vi "Generate Simulated Data.vi"(6 "Acquisition":refnum<queue>, 8 "error in (no error)":errorcluster, 10 "Longueur d'onde":dbl) -> (0 "error out":errorcluster, 2 "Data Out":variant[](array[variant]), 3 "Disconnected":bool=TRUE)   [LabVIEW 2022 SP3, in "Acquisition.lvlib"]
doc: "Generates sample waveforms according to the signal type in the HW Config input."
uses:
  Acquisition.lvlib
  support/Message Queue/Message Cluster.ctl
  <vilib>/DAQmx/write.llb/DAQmx Write (Digital 1D Bool NChan 1Samp 1Line).vi
  <vilib>/numeric/Random Number (Range) U64.vi
  <vilib>/DAQmx/read.llb/DAQmx Read (Analog 1D Wfm NChan NSamp).vi
  <vilib>/Analysis/baseanly.llb/Mean (DBL).vi
  <vilib>/numeric/sub_Random U32.vi
  <vilib>/DAQmx/create/channels.llb/DAQmx Create Channel (DO-Digital Output).vi
  <vilib>/DAQmx/miscellaneous.llb/DAQmx Fill In Error Info.vi
  <vilib>/DAQmx/create/channels.llb/DAQmx Create Channel (AI-Voltage-Basic).vi
  <vilib>/DAQmx/configure/timing.llb/DAQmx Timing (Sample Clock).vi
  support/Message Queue/Enqueue Message (Single).vi
  GlobalVariable/GlobalPowerByTime.vi
  GlobalVariable/GlobalSet0.vi
  GlobalVariable/GlobalPosYbyTime.vi
  GlobalVariable/GlobalPosXbyTime.vi
  GlobalVariable/GlobalProfileByTime.vi
  GlobalVariable/Globalt0.vi
  GlobalVariable/GlobalTimeStep.vi
  <vilib>/gmath/interp.llb/Create Mesh Grid (2D) (x,y arrays).vi
  <vilib>/Analysis/2dsp.llb/2D Convolution (DBL).vi
  <vilib>/Analysis/NI_AALBase.lvlib
  support/Message Queue/Message Queue.lvlib
  <vilib>/gmath/NI_Gmath.lvlib
  <vilib>/Analysis/NI_AALPro.lvlib
  <resource>/objmgr/daqmx.rc
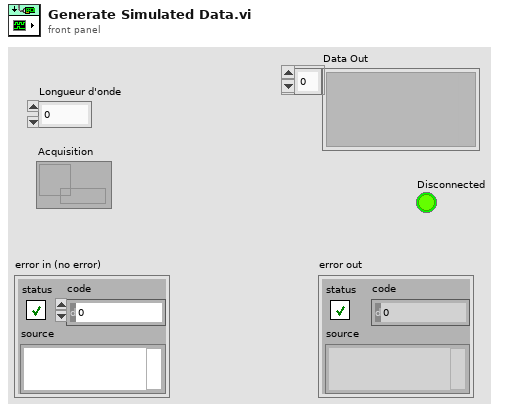
[diagram p1: front panel]
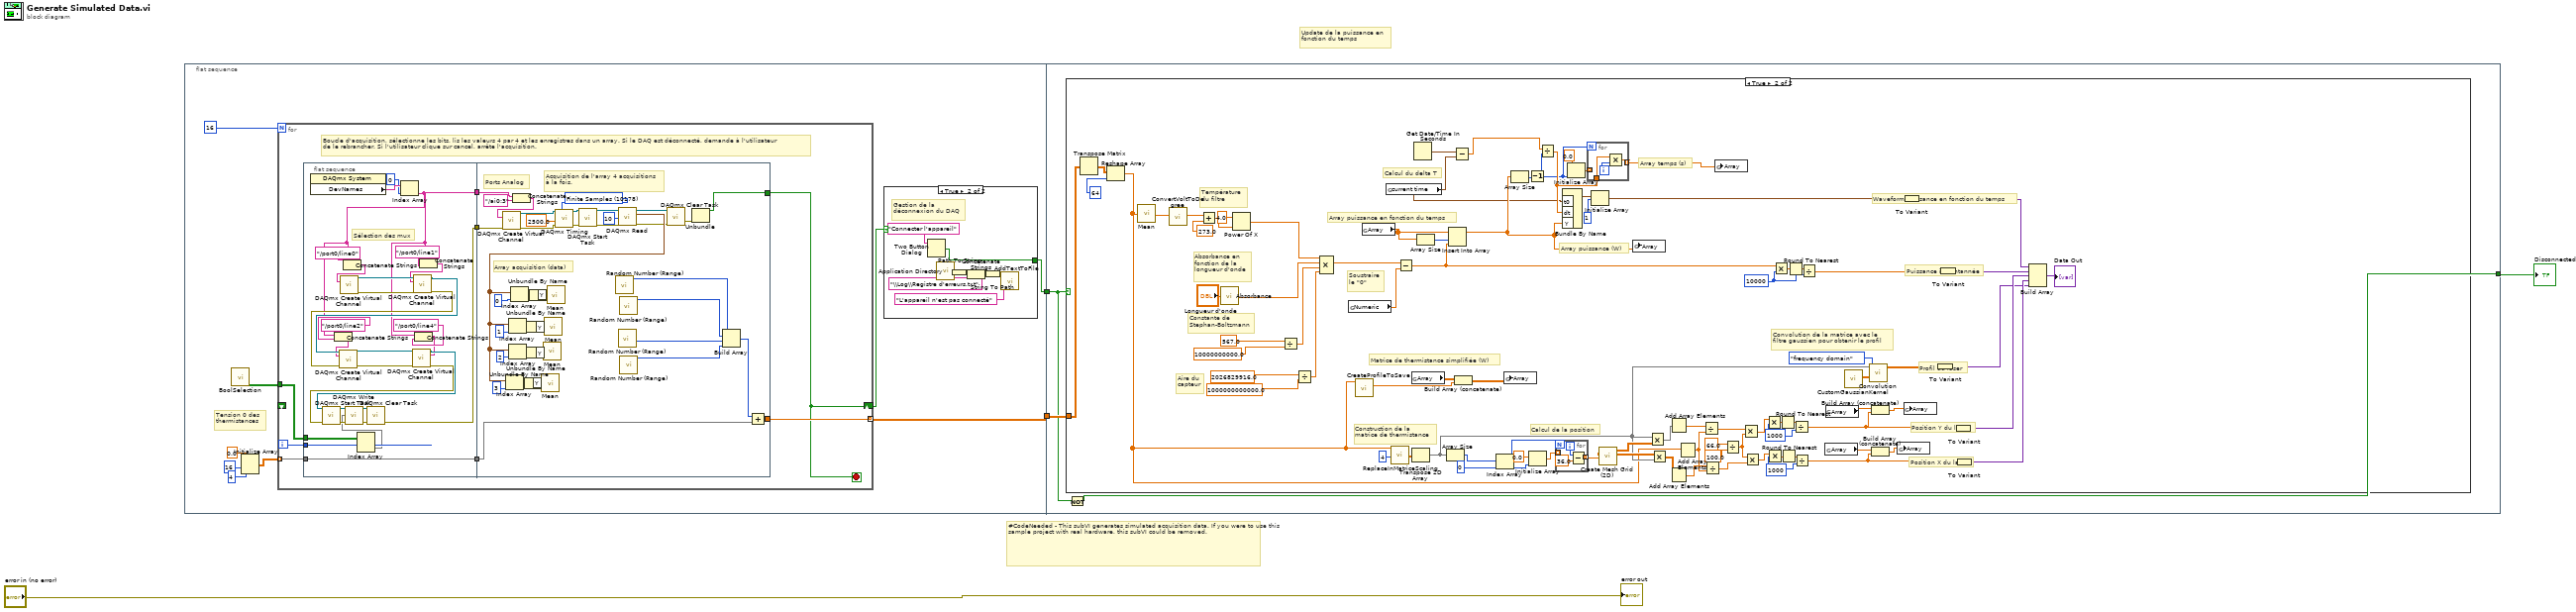
[diagram p0: block diagram]
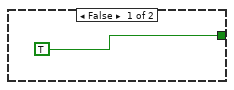
[diagram p2: hidden frame]
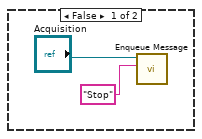
[diagram p3: hidden frame]
diagram:
  # "Update de la puissance en\nfonction du temps"
  # "#CodeNeeded - This subVI generates simulated acquisition data. If you were to use this sample project with real hardware, this subVI could be removed."
  n1 = flat-sequence {
    tunnel: [w11] -> w3
    tunnel: [w10] -> w2
    tunnel: w3 -> [w98]
    tunnel: w2 -> [w97]
    tunnel: [w96] -> w1
    frame #0 {
      # "Tension 0 des \nthermistances"
      n2 = call "BoolSelection.vi"() -> ("BoolSelection"=w12:bool[][])  [unwired: 11 in]
      n3 = Initialize Array(0.0 ("element"), 16 ("dimension size"), 4 ("dimension size")) -> (w6:dbl[][])
      n4 = for {
        N: 16 -> [_]
        tunnel: w12 -> [w28]
        tunnel: w6 -> [w26] mode=indexing
        tunnel: [w25] -> w11 mode=indexing
        shift-right: [w24] -> w5
        shift-left: _ -> [_]
        i -> [w29]
        stop <- w24 stop-if-true
        # "Boucle d'acquisition, sélectionne les bits, lis les valeurs 4 par 4 et les enregistres dans un array. Si le DAQ est déconnecté, demande à l'utilisateur \nde le rebrancher. Si l'utilisateur clique sur cancel, arrête l'acquisition."
        n5 = flat-sequence {
          tunnel: w29 -> [w44]
          tunnel: [w55] -> w30
          tunnel: w28 -> [w43]
          tunnel: [w42] -> w27
          tunnel: w26 -> [w42]
          tunnel: [w31] -> w23
          tunnel: w30 -> [w87]
          tunnel: w27 -> [w62]
          tunnel: [w64] -> w25
          tunnel: [w69] -> w24
          tunnel: w23 -> [w59]
          frame #0 {
            # "Sélection des mux"
            n6 = property class="DAQmx System"() -> ("DevNames"=w41:tag[])  [unwired: 2 in, 2 out]
            n7 = Index Array(array=w43, index (row)=w44) -> (element=w56:bool[])  [unwired: 1 in]
            n8 = Index Array(array=w41, index=0) -> (element=w31:tag)
            n9 = Concatenate Strings(w31, "/port0/line2" ("string")) -> (w34:string)
            n10 = Concatenate Strings(w31, "/port0/line0" ("string")) -> (w39:string)
            n11 = call-poly <vilib>:"DAQmx Create Virtual Channel.vi"("lines"=w39) -> ("task out"=w51:refnum<k21>, "error out"=w52:errorcluster)  [unwired: 13 in]
            n12 = Concatenate Strings(w31, "/port0/line4" ("string")) -> (w32:string)
            n13 = Concatenate Strings(w31, "/port0/line1" ("string")) -> (w36:string)
            n14 = call-poly <vilib>:"DAQmx Create Virtual Channel.vi"("task in"=w51, "lines"=w36, "error in"=w52) -> ("task out"=w50:refnum<k21>, "error out"=w49:errorcluster)  [unwired: 11 in]
            n15 = call-poly <vilib>:"DAQmx Create Virtual Channel.vi"("task in"=w50, "lines"=w34, "error in"=w49) -> ("task out"=w47:refnum<k21>, "error out"=w48:errorcluster)  [unwired: 11 in]
            n16 = call-poly <vilib>:"DAQmx Create Virtual Channel.vi"("task in"=w47, "lines"=w32, "error in"=w48) -> ("task out"=w46:refnum<k21>, "error out"=w45:errorcluster)  [unwired: 11 in]
            n17 = call <vilib>:"DAQmx Start Task.vi"("task/channels in"=w46, "error in"=w45) -> ("task out"=w57:refnum<k21>, "error out"=w58:errorcluster)  [unwired: 12 in]
            n18 = call-poly <vilib>:"DAQmx Write.vi"("task/channels in"=w57, "data"=w56, "error in"=w58) -> ("task out"=w54:refnum<k21>, "error out"=w53:errorcluster)  [unwired: 10 in, 1 out]
            n19 = call <vilib>:"DAQmx Clear Task.vi"("task in"=w54, "error in"=w53) -> ("error out"=w55:errorcluster)  [unwired: 13 in]
          }
          frame #1 {
            w89 = 10178 items=["Finite Samples"=10178, "Continuous Samples"=10123, "Hardware Timed Single Point"=12522] ("sample mode")
            # "Ports Analog"
            # "Array acquisition (data)"
            # "Acquisition de l'array 4 acquisitions\nà la fois."
            n20 = Concatenate Strings(w59, "/ai0:3" ("string")) -> (w60:string)
            n21 = call-poly <vilib>:"DAQmx Create Virtual Channel.vi"("physical channels"=w60, "error in"=w87) -> ("task out"=w94:refnum<k21>, "error out"=w93:errorcluster)  [unwired: 12 in]
            n22 = call-poly <vilib>:"DAQmx Timing.vi"("task/channels in"=w94, "sample mode"=w89, "rate"=2500.0, "error in"=w93) -> ("task out"=w90:refnum<k21>, "error out"=w91:errorcluster)  [unwired: 10 in]
            n23 = call <vilib>:"DAQmx Start Task.vi"("task/channels in"=w90, "error in"=w91) -> ("task out"=w92:refnum<k21>, "error out"=w95:errorcluster)  [unwired: 12 in]
            n24 = call-poly <vilib>:"Random Number (Range).vi"() -> ("number"=w67:u64)  [unwired: 11 in]
            n25 = call-poly <vilib>:"Random Number (Range).vi"() -> ("number"=w65:u64)  [unwired: 11 in]
            n26 = call-poly <vilib>:"DAQmx Read.vi"("task/channels in"=w92, "number of samples per channel"=10, "error in"=w95) -> ("task out"=w71:refnum<k21>, "data"=w80:waveform(dbl)[], "error out"=w70:errorcluster)  [unwired: 10 in]
            n27 = Index Array(array=w80, index=3) -> (element=w76:waveform(dbl))
            n28 = Index Array(array=w80, index=1) -> (element=w78:waveform(dbl))
            n29 = Index Array(array=w80, index=2) -> (element=w77:waveform(dbl))
            n30 = Index Array(array=w80, index=0) -> (element=w79:waveform(dbl))
            n31 = Unbundle By Name(w76) -> ("Y"=w72:dbl[])
            n32 = Unbundle By Name(w78) -> ("Y"=w74:dbl[])
            n33 = Unbundle By Name(w77) -> ("Y"=w73:dbl[])
            n34 = Unbundle By Name(w79) -> ("Y"=w75:dbl[])
            n35 = call-poly <vilib>:"Mean.vi"("X"=w72) -> ()  [unwired: 2 out]
            n36 = call-poly <vilib>:"Mean.vi"("X"=w73) -> ()  [unwired: 2 out]
            n37 = call-poly <vilib>:"Mean.vi"("X"=w74) -> ()  [unwired: 2 out]
            n38 = call-poly <vilib>:"Mean.vi"("X"=w75) -> ()  [unwired: 2 out]
            n39 = call-poly <vilib>:"Random Number (Range).vi"() -> ("number"=w68:u64)  [unwired: 11 in]
            n40 = call-poly <vilib>:"Random Number (Range).vi"() -> ("number"=w66:u64)  [unwired: 11 in]
            n41 = call <vilib>:"DAQmx Clear Task.vi"("task in"=w71, "error in"=w70) -> ("error out"=w85:errorcluster)  [unwired: 13 in]
            n42 = Unbundle(w85) -> ("status"=w69:bool)  [unwired: 2 out]
            n43 = Build Array(w67, w68, w65, w66) -> (w63:u64[])
            n44 = Add(x=w63, y=w62) -> (x+y=w64:dbl[])
          }
        }
      }
      n45 = case shown="True" w5 {
        tunnel: [TRUE w22] -> w10
        frame False {
        }
        frame True {
          # "Gestion de la \ndéconnexion du DAQ"
          n46 = Two Button Dialog(message="Connecter l'appareil") -> (T button?=w22:bool)  [unwired: 2 in]
          n47 = call <vilib>:"Application Directory.vi"() -> ("Application Directory"=w19:path)
          n48 = Path To String(path=w19) -> (string=w20:string)
          n49 = Concatenate Strings(w20, "\\Log\\Registre d'erreurs.txt") -> (w21:string)
          n50 = String To Path(string=w21) -> (path=w17:path)
          n51 = call "AddTextToFile.vi"("Ajouter du texte"="L'appareil n'est pas connecté", "Fichier"=w17) -> ()  [unwired: 10 in]
        }
      }
    }
    frame #1 {
      n52 = case shown="True" w97 {
        tunnel: w98 -> [_ w122]
        frame False {
          n53 = call-poly "Enqueue Message.vi"("Message"="Stop", "Message Queue"="Acquisition") -> ()  [unwired: 8 in, 2 out]
        }
        frame True {
          w136 = 1000
          w140 = 1000
          w146 = 10000
          # "Calcul du delta T"
          # "Matrice de thermistance simplifiée (W)"
          # "Soustraire\nle \"0\""
          # "Constante de \nStephan-Boltzmann"
          # "Absorbance en\nfonction de la \nlongueur d'onde"
          # "Température \ndu filtre"
          # "Aire du\ncapteur"
          # "Calcul de la position"
          # "Construction de la \nmatrice de thermistance"
          # "Position X du laser"
          # "Position Y du laser"
          # "Profil du laser"
          # "Puissance instantannée"
          # "Waveform puissance en fonction du temps"
          # "Array puissance (W)"
          # "Array temps (s)"
          # "Convolution de la matrice avec le \nfiltre gaussien pour obtenir le profil"
          # "Array puissance en fonction du temps"
          n54 = Transpose Matrix(1:w122) -> (0:w123:dbl[][])
          n55 = Reshape Array(w123, 64 ("dimension size")) -> (w117:dbl[])
          n56 = call-poly <vilib>:"Mean.vi"("X"=w117) -> ("mean"=w130:dbl)  [unwired: 1 out]
          n57 = call "ConvertVoltToDegree.vi"("Tension"=w130) -> ("Température"=w129:dbl)  [unwired: 10 in]
          n58 = Add(x=w129, y=273.0) -> (x+y=w175:dbl)
          n59 = call "Absorbance.vi"("Longueur d'onde"="Longueur d'onde") -> ("absorbance"=w126:dbl)  [unwired: 10 in]
          n60 = Power Of X(1:w175, 2:4.0 ("y")) -> (0:w125:dbl)
          n61 = Divide(x=567.0, y=10000000000.0) -> (x/y=w127:dbl)
          n62 = Divide(x=2026829916.0, y=1000000000000.0) -> (x/y=w128:dbl)
          n63 = Compound Arithmetic op=MULTIPLY(w125, w126, w127, w128) -> (w121:dbl)
          n64 = global read "GlobalSet0.vi" "Numeric"() -> (w120:dbl)
          n65 = call "CreateProfileToSave.vi"("Input Array"=w117) -> ("Ouput array"=w107:dbl[])  [unwired: 10 in]
          n66 = global read "GlobalPowerByTime.vi" "Array"() -> (w187:dbl[])
          n67 = global read "Globalt0.vi" "current time"() -> (w102:timestamp)
          n68 = call "ReplaceInMatriceScaling.vi"("Input Scaling"=4, "Input Array"=w117) -> ("Output Array"=w182:dbl[][])  [unwired: 9 in]
          n69 = Subtract(x=w121, y=w120) -> (x-y=w119:dbl)
          n70 = global read "GlobalProfileByTime.vi" "Array"() -> (w106:dbl[][])
          n71 = Transpose 2D Array(2D array=w182) -> (transposed array=w118:dbl[][])
          n72 = Get Date/Time In Seconds() -> (seconds since 1Jan1904=w103:timestamp)
          n73 = Array Size(array=w187) -> (size(s)=w186:i32)
          n74 = Array Size(array=w118) -> (size(s)=w169:i32[])
          n75 = Insert Into Array(array=w187, index=w186, new element=w119) -> (w116:dbl[])
          n76 = Subtract(x=w103, y=w102) -> (x-y=w101:dbl)
          n77 = Build Array (concatenate)(w106, w107) -> (w108:dbl[][])
          n78 = Index Array(array=w169, index=0) -> (element=w164:i32)
          n79 = global write "GlobalProfileByTime.vi" "Array"(w108) -> ()
          n80 = Array Size(array=w116) -> (size(s)=w105:i32)
          n81 = Decrement(x=w105) -> (x-1=w104:i32)
          n82 = Initialize Array(0.0 ("element"), w164) -> (w166:dbl[])
          n83 = Divide(x=w101, y=w104) -> (x/y=w180:dbl)
          n84 = for {
            N: w164 -> [_]
            tunnel: w166 -> [_] mode=indexing
            tunnel: [w188] -> w161 mode=indexing
            i -> [w189]
            n85 = Subtract(x=w189, y=36.0) -> (x-y=w188:dbl)
          }
          n86 = Bundle By Name("t0"=w102, "dt"=w180, "Y"=w116) -> (w184:waveform(dbl))  [unwired: 1 in]
          n87 = Initialize Array(0.0 ("element"), w104) -> (w178:dbl[])
          n88 = for {
            N: w104 -> [_]
            tunnel: w180 -> [w192]
            tunnel: w178 -> [_] mode=indexing
            tunnel: [w191] -> w115 mode=indexing
            i -> [w193]
            n89 = Multiply(x=w192, y=w193) -> (x*y=w191:dbl)
          }
          n90 = Initialize Array(w184, 1) -> (w150:waveform(dbl)[])
          n91 = call-poly <vilib>:"Create Mesh Grid (2D).vi"("y domain"=w161, "x domain"=w161) -> ("Y"=w160:dbl[][], "X"=w165:dbl[][])  [unwired: 7 in, 1 out]
          n92 = global write "GlobalPowerByTime.vi" "Array"(w116) -> ()
          n93 = Multiply(x=w118, y=w165) -> (x*y=w163:dbl[][])
          n94 = Multiply(x=w160, y=w118) -> (x*y=w159:dbl[][])
          n95 = Add Array Elements(numeric array=w163) -> (sum=w162:dbl)
          n96 = Add Array Elements(numeric array=w159) -> (sum=w158:dbl)
          n97 = Add Array Elements(numeric array=w117) -> (sum=w157:dbl)
          n98 = Divide(x=w162, y=w157) -> (x/y=w155:dbl)
          n99 = Divide(x=w158, y=w157) -> (x/y=w156:dbl)
          n100 = global write "GlobalTimeStep.vi" "Array"(w115) -> ()
          n101 = Divide(x=66.0, y=100.0) -> (x/y=w154:dbl)
          n102 = Multiply(x=w155, y=w154) -> (x*y=w137:dbl)
          n103 = Multiply(x=w154, y=w156) -> (x*y=w133:dbl)
          n104 = Multiply(x=w137, y=w140) -> (x*y=w139:dbl)
          n105 = Multiply(x=w133, y=w136) -> (x*y=w135:dbl)
          n106 = Multiply(x=w119, y=w146) -> (x*y=w147:dbl)
          n107 = Round To Nearest(number=w139) -> (nearest integer value=w138:dbl)
          n108 = Round To Nearest(number=w135) -> (nearest integer value=w134:dbl)
          n109 = Round To Nearest(number=w147) -> (nearest integer value=w145:dbl)
          n110 = Divide(x=w138, y=w140) -> (x/y=w109:dbl)
          n111 = Divide(x=w134, y=w136) -> (x/y=w113:dbl)
          n112 = Divide(x=w145, y=w146) -> (x/y=w141:dbl)
          n113 = global read "GlobalPosYbyTime.vi" "Array"() -> (w114:dbl[])
          n114 = global read "GlobalPosXbyTime.vi" "Array"() -> (w110:dbl[])
          n115 = call "CustomGaussianKernel.vi"() -> ("array"=w177:dbl[][])  [unwired: 11 in]
          n116 = call-poly <vilib>:"Convolution.vi"("algorithm"=enum32{"direct", "frequency domain"}."frequency domain", "Y"=w177, "X"=w118) -> ("X * Y"=w131:dbl[][])  [unwired: 7 in, 1 out]
          n117 = Build Array (concatenate)(w110, w109) -> (w111:dbl[])
          n118 = Build Array (concatenate)(w114, w113) -> (w112:dbl[])
          n119 = global write "GlobalPosYbyTime.vi" "Array"(w112) -> ()
          n120 = To Variant(anything=w150) -> (Variant=w149:variant)
          n121 = global write "GlobalPosXbyTime.vi" "Array"(w111) -> ()
          n122 = To Variant(anything=w131) -> (Variant=w132:variant)
          n123 = To Variant(anything=w141) -> (Variant=w142:variant)
          n124 = To Variant(anything=w109) -> (Variant=w143:variant)
          n125 = To Variant(anything=w113) -> (Variant=w144:variant)
          n126 = Build Array(w149, w142, w143, w144, w132) -> (→"Data Out":variant[])
        }
      }
      n127 = Not(x=w97) -> (.not. x?=w96:bool)
    }
  }
  "error out" <- "error in (no error)"
  "Disconnected" <- w1
